vi "displayConfigurableElements.vi"(11 "ConfigurationThisComponent in":refnum<class "ConfigurationThisComponent.lvclass">) -> (3 "ConfigurationThisComponent out":refnum<class "ConfigurationThisComponent.lvclass">)   [LabVIEW 2013, in "ConfigurationThisComponent.lvclass"]
uses:
  ConfigurationThisComponent.lvclass
  <userlib>/Common/ILC/Configuration/ILCSerial.ctl
  <userlib>/Common/SerialProtocols/Configuration/SerialConfig.ctl
  <userlib>/Common/SerialProtocols/Configuration/SerialProtocol.ctl
  <userlib>/Common/SerialProtocols/Configuration/ProtocolParameters.ctl
  <userlib>/Common/SerialProtocols/Configuration/SerialMessageParameters.ctl
  <userlib>/Common/Devices/DistanceGauge/Config/DistanceGauge.ctl
  <userlib>/Common/Devices/DistanceGauge/Config/ChannelsToRead.ctl
  <userlib>/Common/Devices/ForceSensorCalculator/Config/ForceSensorCalculator.ctl
  <userlib>/Common/Devices/ForceSensorCalculator/Config/BridgeResistors.ctl
  Configuration/SystemController.ctl
  Configuration/PIDGains.ctl
  <userlib>/Common/Devices/StepperMotor/Config/StepperMotor.ctl
  <userlib>/Common/Devices/EncoderConverter/Config/EncoderConverter.ctl
  Configuration/Thermocouple.ctl
  Configuration/MotorOverheatTemperature.ctl
  <userlib>/Common/ILC/Configuration/ILCADC.ctl
  <userlib>/Common/ILC/Configuration/InputChannels.ctl
  <userlib>/Common/ILC/Configuration/ScanRate_Hz_MultichannelOptions.ctl
  Configuration/StiffnessMonitor.ctl
  <userlib>/Common/SerialProtocols/SerialProtocols.lvlib
  <userlib>/Common/ILC/Configuration/ILCConfiguration.lvlib
  <userlib>/Common/Devices/DistanceGauge/DistanceGauge.lvlib
  <userlib>/Common/Devices/ForceSensorCalculator/ForceSensorCalculator.lvlib
  <userlib>/Common/Devices/StepperMotor/StepperMotor.lvlib
  <userlib>/Common/Devices/EncoderConverter/EncoderConverter.lvlib
panel:
  in  "ctrlRefArrayUsrEvnt":refnum<user-event>
  in  "ConfigTab":T1(tab)
  in  "ILCSerial":T2={"Serial"={"Serial Protocol"=enum."RS485", "Protocol Parameters"={"VISA resource name"="", "Baud Rate"=9600, "Data Bits"=8, "Parity"=enum."None", "Flow Control"=0, "Stop Bits"=10, "Timeout (ms)"=10000}, "Serial Message Parameters"={"Byte Count"=200, "Enable Termination Character"=FALSE, "Termination Char"=200}}} {"Serial"."Serial Message Parameters"."Termination Char" format="%x"; "Serial"."Protocol Parameters"."Stop Bits" items=["1.0"=10, "1.5"=15, "2.0"=20]; "Serial"."Protocol Parameters"."Flow Control" items=["None", "XON/XOFF", "RTS/CTS", "XON/XOFF & RTS/CTS", "DTR/DSR", "XON/XOFF & DTR/DSR"]; "Serial"."Protocol Parameters"."Data Bits" min=5 max=8 step=1}
  in  "ILCADC":T7={"Input Channels"=enum."Channel 0", "Scan Rate (Hz) "=enum."50", "PGA Gain Coefficient"=0, "Reference Voltage Vref"=0.0, "Nominal Input Range in Counts"=128, "Preamplifier Gain"=0, "Conversion Settling Cycles"=0} {"Conversion Settling Cycles" min=1; "Preamplifier Gain" min=1; "Nominal Input Range in Counts" min=128; "Reference Voltage Vref" min=-10.0 max=10.0 format="%.3f"; "PGA Gain Coefficient" max=7}
  in  "DistanceGauge":T10={"Serial"={"Serial Protocol"=enum."RS485", "Protocol Parameters"={"VISA resource name"="", "Baud Rate"=9600, "Data Bits"=8, "Parity"=enum."None", "Flow Control"=0, "Stop Bits"=10, "Timeout (ms)"=10000}, "Serial Message Parameters"={"Byte Count"=200, "Enable Termination Character"=FALSE, "Termination Char"=200}}, "Channels To Read"=[]} {"Serial"."Serial Message Parameters"."Termination Char" format="%x"; "Serial"."Protocol Parameters"."Stop Bits" items=["1.0"=10, "1.5"=15, "2.0"=20]; "Serial"."Protocol Parameters"."Flow Control" items=["None", "XON/XOFF", "RTS/CTS", "XON/XOFF & RTS/CTS", "DTR/DSR", "XON/XOFF & DTR/DSR"]; "Serial"."Protocol Parameters"."Data Bits" min=5 max=8 step=1}
  in  "ForceSensorCalculator":T12={"Capacity"=5.0, "Sensitivity"=0.001, "Bridge Resistors"={"R1"=1.0, "R2"=1.0}} {"Bridge Resistors"."R2" min=1.0 max=5000000.0 format="%.1f"; "Bridge Resistors"."R1" min=1.0 max=5000000.0 format="%.1f"; "Sensitivity" min=0.001 max=5000.0 format="%.5f"; "Capacity" min=1.0 max=5000000.0 format="%.4f"}
  in  "EncoderConverter":T14 {"Distance Per Count" format="%.3f"}
  in  "Thermocouple":T15={"Thermocouple Conversion"=274.15, "Motor Overheat Temperature"=274.15, "Ambient Temperature"=274.15} {"Ambient Temperature" min=-26.850000000000023 max=573.15 format="%.1f"; "Motor Overheat Temperature" min=-26.850000000000023 max=573.15 format="%.1f"; "Thermocouple Conversion" min=274.15 max=5000273.15 format="%.5f"}
  in  "SystemController":T17={"PID Gains"={"Proportional Gain (Kc)"=1.0, "Integral Time (Ti, min)"=0.01, "Derivative Time (Td, min)"=0.0}, "Force Error In Range Limit"=5000.0} {"PID Gains"."Derivative Time (Td, min)" format="%.3f"; "PID Gains"."Integral Time (Ti, min)" format="%.3f"; "PID Gains"."Proportional Gain (Kc)" format="%.3f"; "Force Error In Range Limit" min=0.01 max=5000.0 format="%.2f"}
  in  "StepperMotor":T19={"Maximum Step Rate"=5000000.0} {"Maximum Step Rate" min=1.0 max=4000.0 format="%.3f"}
  in  "StiffnessMonitor":T20={"Stiffness Lower Limit"=2000000.0} {"Stiffness Lower Limit" min=1000.0 max=100000000.0 format="%.2f"}
  # "Gain is 2^gain_coefficient"
  # "defined at capacity"
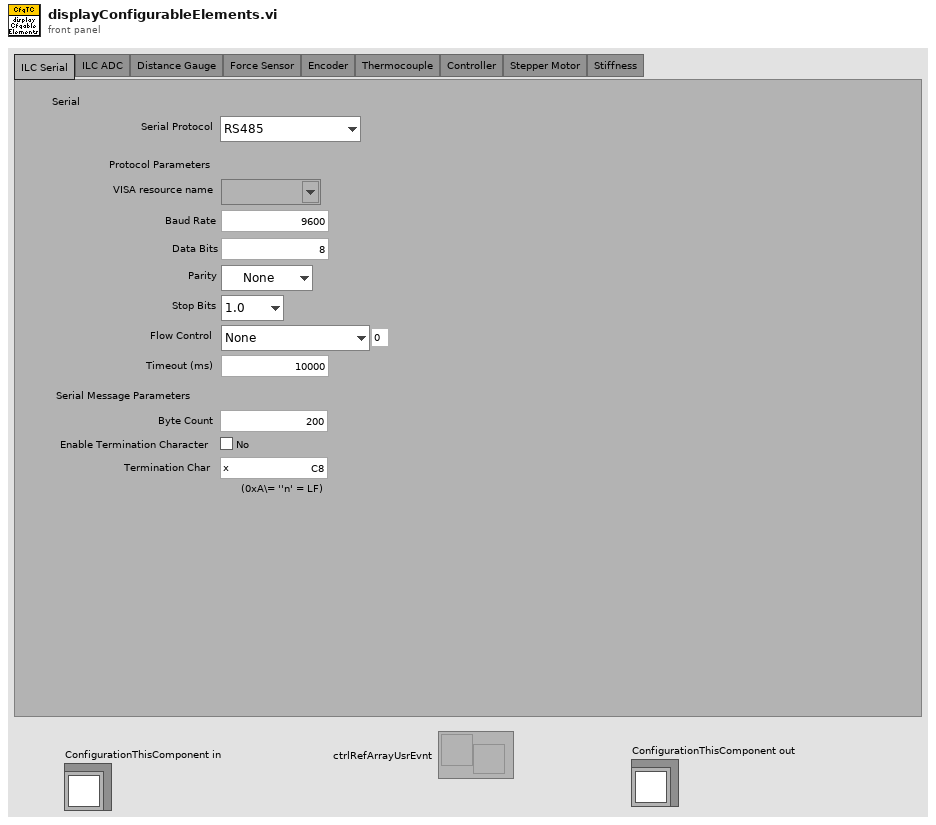
[diagram p1: front panel]
types:
  T1 = enum32{"ILC Serial", "ILC ADC", "Distance Gauge", "Force Sensor", "Encoder", "Thermocouple", "Controller", "Stepper Motor", "Stiffness"}
  T2 = typedef "ILCCommon.lvlib/ILCConfiguration.lvlib/ILCSerial.ctl" = cluster{"Serial":T3}
  T3 = typedef "SerialProtocols.lvlib/SerialConfig.ctl" = cluster{"Serial Protocol":T4, "Protocol Parameters":T5, "Serial Message Parameters":T6}
  T4 = typedef "SerialProtocols.lvlib/SerialProtocol.ctl" = enum16{"RS232", "RS485", "SerialSimulator"}
  T5 = typedef "SerialProtocols.lvlib/ProtocolParameters.ctl" = cluster{"VISA resource name":refnum<visa-resource-name>, "Baud Rate":u32, "Data Bits":u16, "Parity":enum16{"None", "Odd", "Even", "Mark", "Space"}, "Flow Control":u16, "Stop Bits":u16, "Timeout (ms)":u32}
  T6 = typedef "SerialProtocols.lvlib/SerialMessageParameters.ctl" = cluster{"Byte Count":u32, "Enable Termination Character":bool, "Termination Char":u8}
  T7 = typedef "ILCCommon.lvlib/ILCConfiguration.lvlib/ILCADC.ctl" = cluster{"Input Channels":T8, "Scan Rate (Hz) ":T9, "PGA Gain Coefficient":u8, "Reference Voltage Vref":dbl[unit], "Nominal Input Range in Counts":u32, "Preamplifier Gain":u8, "Conversion Settling Cycles":u16}
  T8 = typedef "ILCCommon.lvlib/ILCConfiguration.lvlib/InputChannels.ctl" = enum16{"Channel 0", "3 Channels", "5 Channels"}
  T9 = typedef "ILCCommon.lvlib/ILCConfiguration.lvlib/ScanRate_Hz_MultichannelOptions.ctl" = enum16{"50", "60", "100", "120", "200", "240", "300", "400", "480", "600", "1200", "2400", "4800"}
  T10 = typedef "DistanceGauge.lvlib/DistanceGauge.ctl" = cluster{"Serial":T3, "Channels To Read":T11}
  T11 = typedef "DistanceGauge.lvlib/ChannelsToRead.ctl" = i32[]
  T12 = typedef "ForceSensorCalculator.lvlib/ForceSensorCalculator.ctl" = cluster{"Capacity":dbl[unit], "Sensitivity":dbl[unit], "Bridge Resistors":T13}
  T13 = typedef "ForceSensorCalculator.lvlib/BridgeResistors.ctl" = cluster{"R1":dbl[unit], "R2":dbl[unit]}
  T14 = typedef "EncoderConverter.lvlib/EncoderConverter.ctl" = cluster{"Distance Per Count":dbl[unit]}
  T15 = typedef "Thermocouple.ctl" = cluster{"Thermocouple Conversion":dbl[unit], "Motor Overheat Temperature":T16, "Ambient Temperature":T16}
  T16 = typedef "MotorOverheatTemperature.ctl" = dbl[unit]
  T17 = typedef "SystemController.ctl" = cluster{"PID Gains":T18, "Force Error In Range Limit":dbl[unit]}
  T18 = typedef "PIDGains.ctl" = cluster{"Proportional Gain (Kc)":dbl, "Integral Time (Ti, min)":dbl, "Derivative Time (Td, min)":dbl}
  T19 = typedef "StepperMotor.lvlib/StepperMotor.ctl" = cluster{"Maximum Step Rate":dbl[unit]}
  T20 = typedef "StiffnessMonitor.ctl" = cluster{"Stiffness Lower Limit":dbl[unit]}
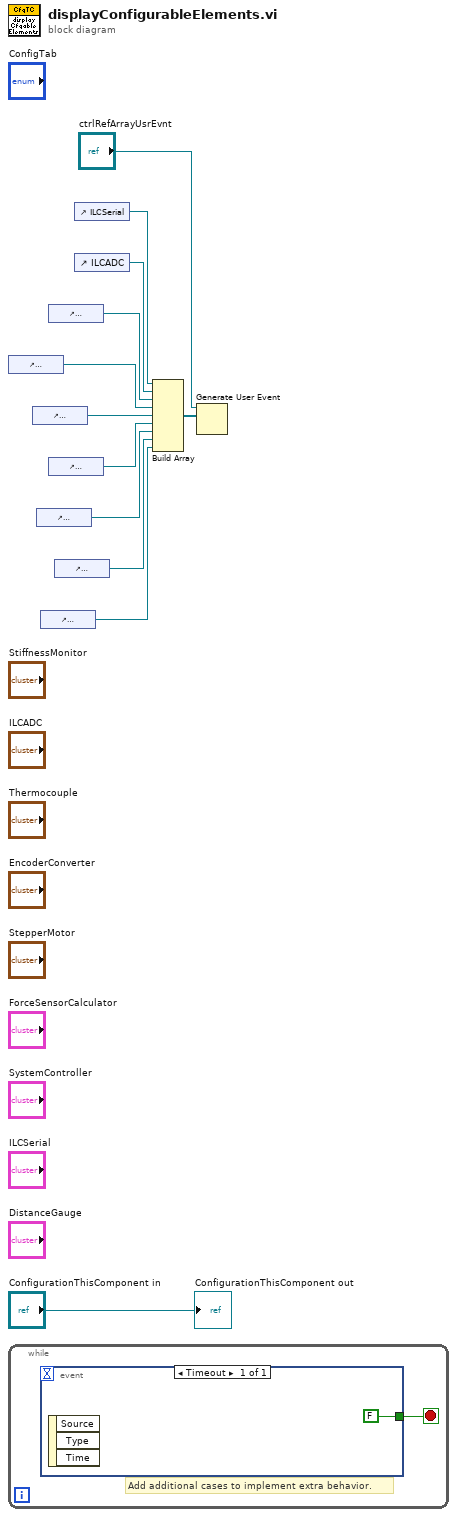
[diagram p0: block diagram]
diagram:
  n1 = control-ref of="ForceSensorCalculator"() -> (w7:refnum<vi>)
  n2 = while {
    stop <- w13 stop-if-true
    # "Add additional cases to implement extra behavior."
    n3 = event shown="[0] Timeout" {
      selector: _ -> [_]
      dyn-events: _ -> [_]
      timeout: _ -> [_]
      tunnel: [FALSE] -> w13
      event Timeout {
        n4 = event-data() -> ()  [unwired: 1 in, 3 out]
      }
    }
  }
  n5 = control-ref of="EncoderConverter"() -> (w6:refnum<vi>)
  n6 = control-ref of="SystemController"() -> (w3:refnum<vi>)
  n7 = control-ref of="StiffnessMonitor"() -> (w1:refnum<vi>)
  n8 = control-ref of="DistanceGauge"() -> (w8:refnum<vi>)
  n9 = control-ref of="Thermocouple"() -> (w5:refnum<vi>)
  n10 = control-ref of="StepperMotor"() -> (w2:refnum<vi>)
  n11 = control-ref of="ILCSerial"() -> (w9:refnum<vi>)
  n12 = control-ref of="ILCADC"() -> (w4:refnum<vi>)
  n13 = Build Array(w9, w4, w8, w7, w6, w5, w3, w2, w1) -> (w12:refnum<vi>[])
  n14 = Generate User Event(user event="ctrlRefArrayUsrEvnt", event data cluster=w12) -> ()  [unwired: 2 in, 2 out]
  "ConfigurationThisComponent out" <- "ConfigurationThisComponent in"
